vi "Happy Number.vi"(8 "Error In":errorcluster, 11 "Numeric":i32) -> (0 "Error Out":errorcluster, 3 "String":string)   [LabVIEW 2024]
doc: "This VI find if the input is happy or non happy number. See BD desciption for more details"
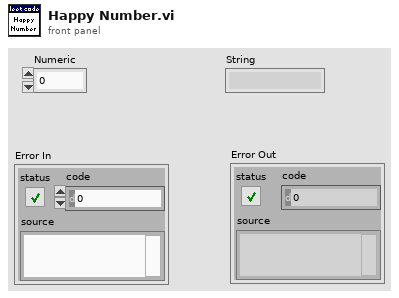
[diagram p1: front panel]
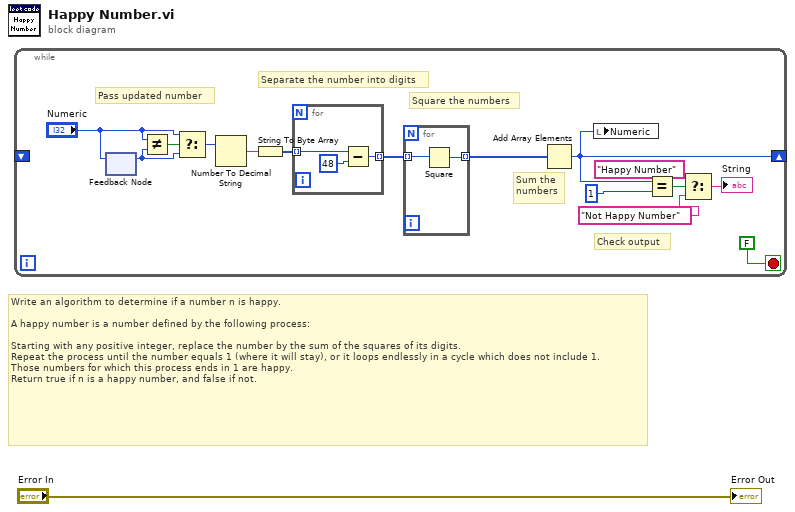
[diagram p0: block diagram]
diagram:
  # "Write an algorithm to determine if a number n is happy.\n\nA happy number is a number defined by the following process:\n\nStarting with any positive integer, replace the number by the sum of the squares of its digits.\nRepeat the process until the number equals 1 (where it will stay), or it loops endlessly in a cycle which does not include 1.\nThose numbers for which this process ends in 1 are happy.\nReturn true if n is a happy number, and false if not."
  n1 = while {
    shift-right: [w6] -> _
    shift-left: _ -> [_]
    stop <- FALSE stop-if-true
    # "Check output"
    # "Sum the \nnumbers"
    # "Square the numbers"
    # "Separate the number into digits"
    # "Pass updated number"
    n2 = feedback-in #1("Numeric") -> ()
    n3 = feedback #1() -> (w3:i32)  [unwired: 1 in]
    n4 = Not Equal?(x="Numeric", y=w3) -> (x != y?=w5:bool)
    n5 = Select(t="Numeric", s=w5, f=w3) -> (s? t:f=w2:i32)
    n6 = Number To Decimal String(number=w2) -> (decimal integer string=w8:string)  [unwired: 1 in]
    n7 = String To Byte Array(string=w8) -> (unsigned byte array=w9:u8[])
    n8 = for {
      tunnel: w9 -> [w19] mode=indexing
      tunnel: [w17] -> w7 mode=indexing
      n9 = Subtract(x=w19, y=u8 48) -> (x-y=w17:u8)
    }
    n10 = for {
      tunnel: w7 -> [w21] mode=indexing
      tunnel: [w20] -> w10 mode=indexing
      n11 = Square(x=w21) -> (x^2=w20:u8)
    }
    n12 = Add Array Elements(numeric array=w10) -> (sum=w6:u8)
    n13 = local write "Numeric"(w6) -> ()
    n14 = Equal?(x=w6, y=u8 1) -> (x = y?=w14:bool)
    n15 = Select(t="Happy Number" ("String 2"), s=w14, f="Not Happy Number" ("String 2")) -> (s? t:f=→"String":string)
  }
  "Error Out" <- "Error In"
